vi "PH_BlackBox.ProcPeriodic.vi"(0 "i ref in":refnum<vi>, 3 "ms timeout (100)":i32=100, 5 "error in (no error)":errorcluster) -> (14 "i ref out":refnum<vi>, 17 "timed out":bool, 19 "error out":errorcluster)   [LabVIEW 2014, in "PH_BlackBox.lvlib"]
doc: "This method serves to periodically do things like reading values from the HW. Methods that should be executed periodically should be called from THIS methode. Add code here."
uses:
  PH_BlackBox.lvlib
  CS_Core/CSSystem/CSSystemLib/CSSystemLib.lvlib
  PH_Basics/PH_StatusHandler/PH_StatusHandler.lvlib
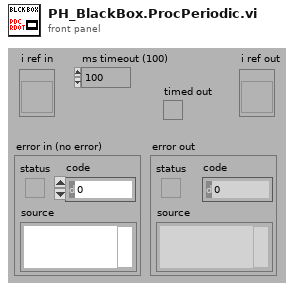
[diagram p1: front panel]
types:
  T1 = typedef "PH_StatusHandler.lvlib/PH_StatusHandler.Status.ctl" = i16
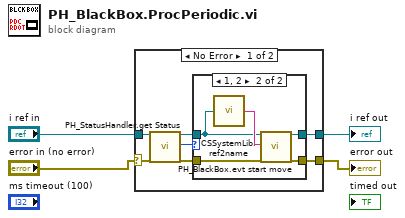
[diagram p0: block diagram]
diagram:
  n1 = case shown="No Error" "error in (no error)" {
    selector: "error in (no error)" -> [w6 w19]
    tunnel: [w11 w19] -> w4
    tunnel: [w10 w20] -> w3
    tunnel: "i ref in" -> [w9 w20]
    frame No Error {
      n2 = call "PH_StatusHandler.get Status.vi"("VI in"=w9, "error in"=w6) -> ("VI out"=w8:refnum<vi>, "Status"=w5:T1, "error out"=w7:errorcluster)  [unwired: 15 in]
      n3 = case shown="1, 2" w5 {
        tunnel: [w12 w18] -> w11
        tunnel: [w13 w17] -> w10
        tunnel: w8 -> [w13 w15]
        tunnel: w7 -> [w12 w14]
        frame Default {
        }
        frame 1, 2 {
          n4 = call "CSSystemLib.ref2name.vi"("obj refnum"=w15) -> ("name"=w16:string)
          n5 = call "PH_BlackBox.evt start move.vi"("i ref in"=w15, "Instance"=w16, "error in (no error)"=w14) -> ("i ref out"=w17:refnum<vi>, "error out"=w18:errorcluster)  [unwired: 15 in]
        }
      }
    }
    frame Error {
    }
  }
  "error out" <- w4
  "i ref out" <- w3
